vi "Triggered Waveform Modifier.vi"(9 "Index":dbl, 10 "Buffer":dbl, 11 "Input Y Values":dbl[](array[numeric])) -> (3 "appended array":dbl[](array[numeric]))   [LabVIEW 2014]
panel:
  # "Triggered Waveform Modifier VI"
  # "Output"
  # "Inputs"
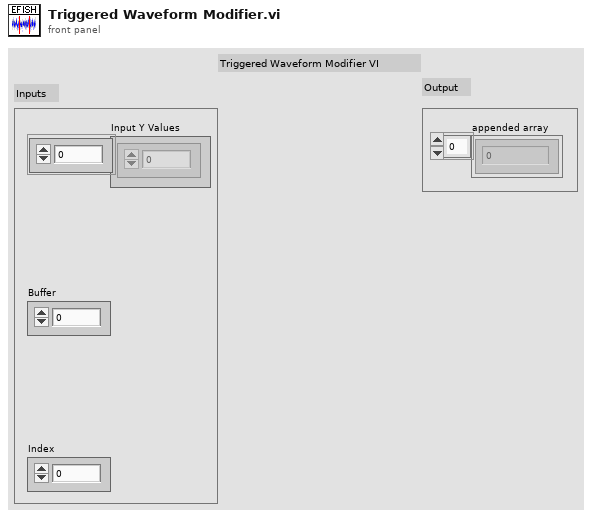
[diagram p1: front panel]
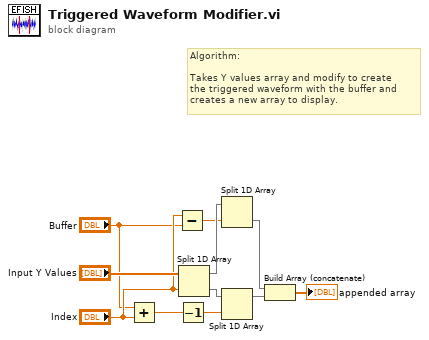
[diagram p0: block diagram]
diagram:
  # "Algorithm:\n\nTakes Y values array and modify to create\nthe triggered waveform with the buffer and\ncreates a new array to display."
  n1 = Add(x="Buffer", y="Index") -> (x+y=w5:dbl)
  n2 = Subtract(x="Index", y="Buffer") -> (x-y=w1:dbl)
  n3 = Decrement(x=w5) -> (x-1=w4:dbl)
  n4 = Split 1D Array(array="Input Y Values", index="Index") -> (first subarray=w10:dbl[], second subarray=w9:dbl[])
  n5 = Split 1D Array(array=w10, index=w1) -> (second subarray=w6:dbl[])  [unwired: 1 out]
  n6 = Split 1D Array(array=w9, index=w4) -> (first subarray=w7:dbl[])  [unwired: 1 out]
  n7 = Build Array (concatenate)(w6, w7) -> (→"appended array":dbl[])
